vi "Read Force Sensor Settings.vi"(8 "error in (no error)":errorcluster, 11 "Boot Loader in":refnum<class "Boot Loader.lvclass">) -> (0 "error out":errorcluster, 2 "Force Sensor Settings":T1={"Reference Voltage Vref"=0.0, "FC1 Force Sensor"={"Capacity"=1.0, "Sensitivity"=0.001}, "FC2 Force Sensor"={"Capacity"=1.0, "Sensitivity"=0.001}} {"FC2 Force Sensor"."Sensitivity" min=0.001 max=5000.0 format="%.4f"; "FC2 Force Sensor"."Capacity" min=1.0 max=5000000.0 format="%.4f"; "FC1 Force Sensor"."Sensitivity" min=0.001 max=5000.0 format="%.4f"; "FC1 Force Sensor"."Capacity" min=1.0 max=5000000.0 format="%.4f"; "Reference Voltage Vref" min=-10.0 max=10.0 format="%.3f"}, 3 "Boot Loader out":refnum<class "Boot Loader.lvclass">)   [LabVIEW 2015, in "Boot Loader.lvclass"]
uses:
  Boot Loader.lvclass
  Typedefs/Force Sensor Settings.ctl
  <userlib>/Common/Devices/ForceSensorCalculator/Config/ForceSensorCalculator.ctl
  Typedefs/FAMT Typedefs.lvlib
  <userlib>/Common/Devices/ForceSensorCalculator/ForceSensorCalculator.lvlib
  Settings/Settings.lvclass
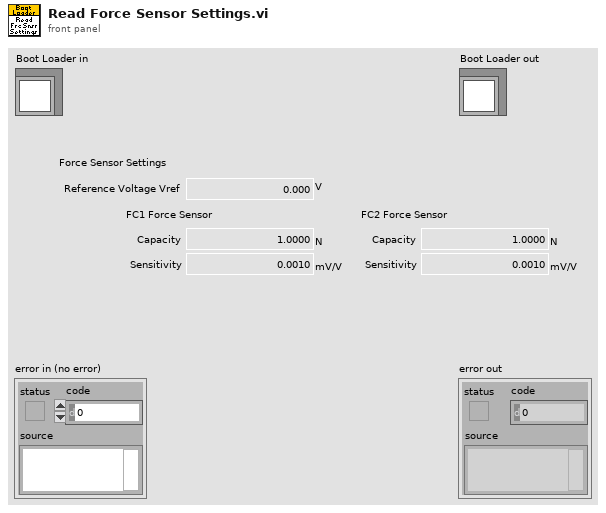
[diagram p1: front panel]
types:
  T1 = typedef "FAMT Typedefs.lvlib/Force Sensor Settings.ctl" = cluster{"Reference Voltage Vref":dbl[unit], "FC1 Force Sensor":T2, "FC2 Force Sensor":T2}
  T2 = typedef "ForceSensorCalculator.lvlib/ForceSensorCalculator.ctl" = cluster{"Capacity":dbl[unit], "Sensitivity":dbl[unit]}
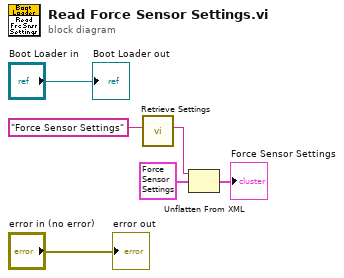
[diagram p0: block diagram]
diagram:
  n1 = call "Retrieve Settings.vi"("configName"="Force Sensor Settings") -> ("xmlConfig"=w3:string)  [unwired: 8 in, 2 out]
  n2 = Unflatten From XML(xml string=w3, type=T1 {"Reference Voltage Vref"=0.0, "FC1 Force Sensor"={"Capacity"=1.0, "Sensitivity"=0.001}, "FC2 Force Sensor"={"Capacity"=1.0, "Sensitivity"=0.001}} ("Force Sensor Settings")) -> (value=→"Force Sensor Settings":T1)  [unwired: 1 in, 1 out]
  "error out" <- "error in (no error)"
  "Boot Loader out" <- "Boot Loader in"
